vi "CmdSet_Cmd_OMAN.vi.bak.vi"(10 "cmd in":string="COLUMS 4096 ROWS 4112 PRESCAN 53 OVERSCAN 62 UTILITY /home/config/SOIAPP/DHE/util.lod TIMING_NORMAL /home/config/SOIAPP/DHE/tim_normal.lod TIMING_FOCUS /home/config/SOIAPP/DHE/tim_focus.lod READOUTMODE 3 MULTEXTEN TRUE HDR /home/config/SOIAPP/sifs.hdr SHOWIMAGE FALSE BINX 1 BINY 1 ENABLEROI FALSE ROIXCENTER 2098 ROIXSIZE 800 ROIYCENTER 2056 ROIYSIZE 400") -> (2 "cmd out":string)   [LabVIEW 2016]
panel:
  in  "bin 2":cluster{"x":i16, "y":i16}
  in  "roi 2":cluster{"xc":i16, "yc":i16, "xl":i16, "yl":i16}
  in  "bin":cluster{"x":i16, "y":i16}
  in  "roi":cluster{"xc":i16, "yc":i16, "xl":i16, "yl":i16}
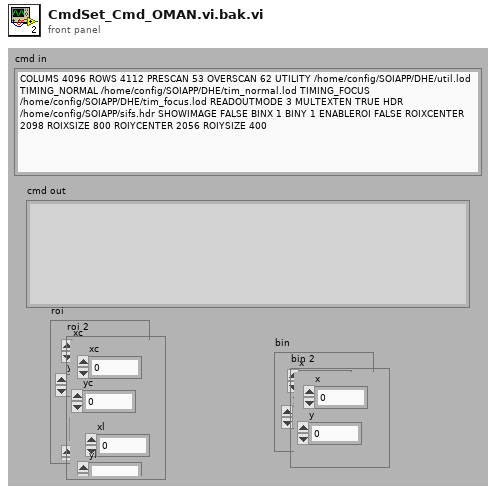
[diagram p1: front panel]
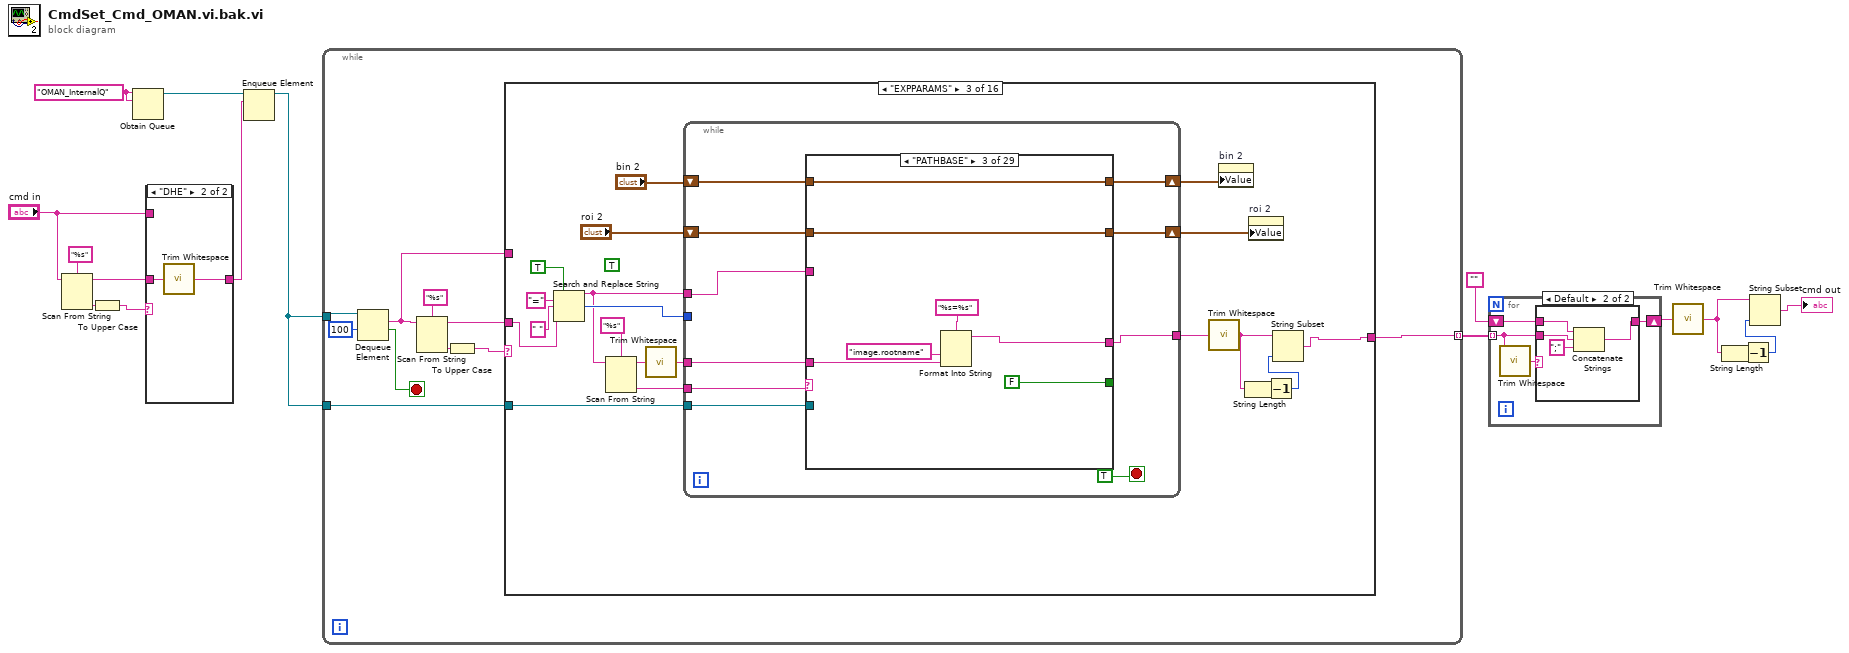
[diagram p0: block diagram]
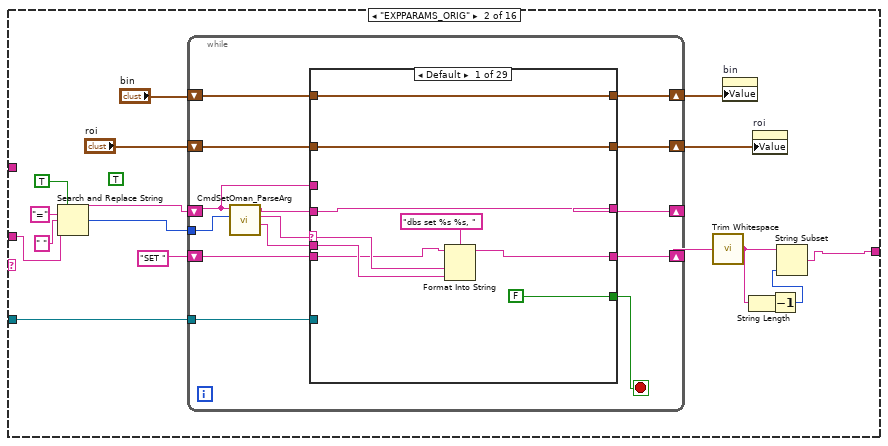
[diagram p4: hidden frame]
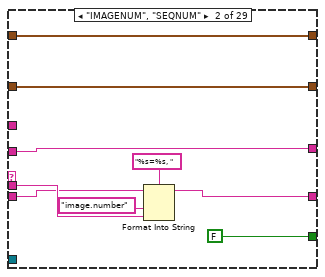
[diagram p5: hidden frame]
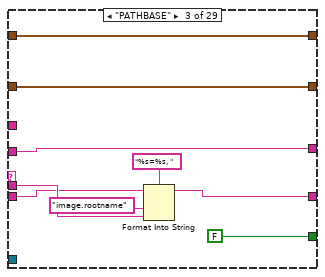
[diagram p6: hidden frame]
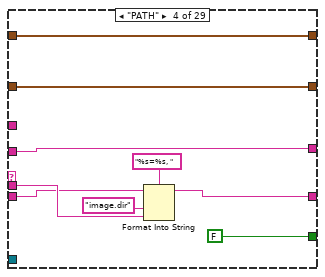
[diagram p7: hidden frame]
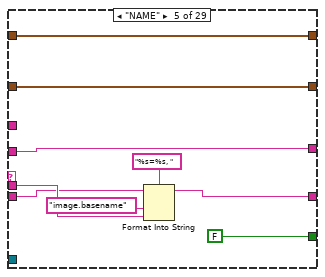
[diagram p8: hidden frame]
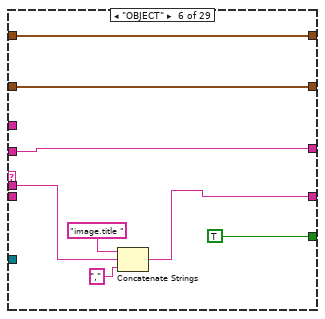
[diagram p9: hidden frame]
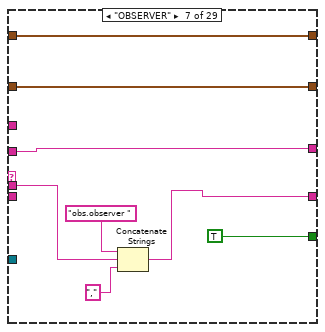
[diagram p10: hidden frame]
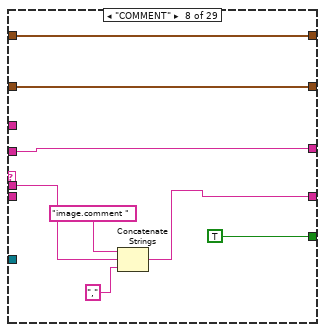
[diagram p11: hidden frame]
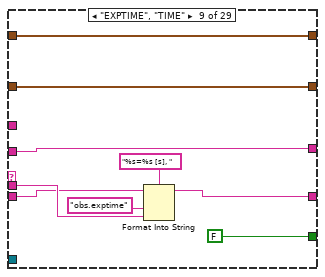
[diagram p12: hidden frame]
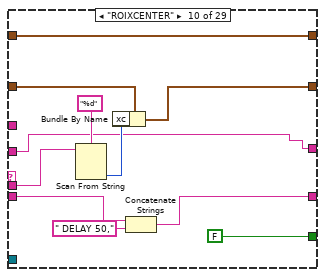
[diagram p13: hidden frame]
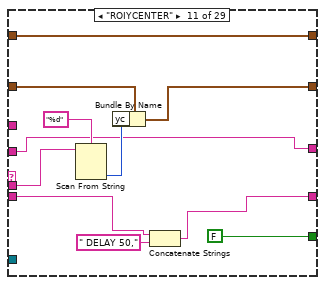
[diagram p14: hidden frame]
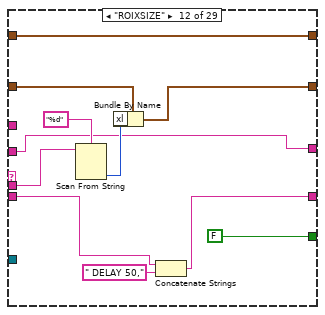
[diagram p15: hidden frame]
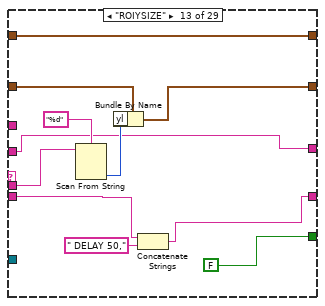
[diagram p16: hidden frame]
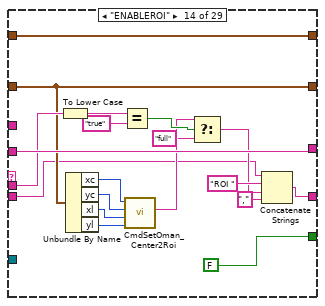
[diagram p17: hidden frame]
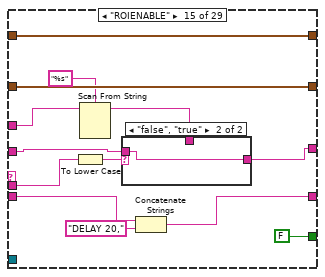
[diagram p18: hidden frame]
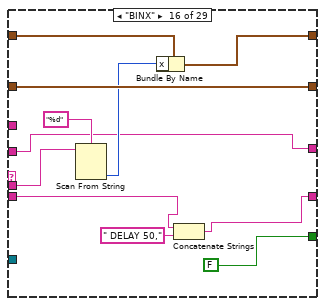
[diagram p20: hidden frame]
diagram:
  w11 = "OMAN_InternalQ" ("name (unnamed)")
  n1 = Scan From String(format string="%s", input string="cmd in") -> (remaining string=w13:string, output 1=w15:string)  [unwired: 2 in, 3 out]
  n2 = To Upper Case(1:w15) -> (0:w14:string)
  n3 = Obtain Queue(name (unnamed)=w11, element data type=w11) -> (queue out=w10:refnum<queue>)  [unwired: 3 in, 2 out]
  n4 = case shown="\"DHE\"" w14 {
    tunnel: w13 -> [_ w19]
    tunnel: [w17 w18] -> w9
    tunnel: "cmd in" -> [w17 _]
    frame Default {
    }
    frame "DHE" {
      n5 = call <vilib>:"Trim Whitespace.vi"("string"=w19) -> ("trimmed string"=w18:string)  [unwired: 1 in]
    }
  }
  n6 = Enqueue Element(queue=w10, element=w9) -> (queue out=w8:refnum<queue>)  [unwired: 1 in, 3 out]
  n7 = while {
    tunnel: w8 -> [w27]
    tunnel: w8 -> [w23]
    tunnel: [w21] -> w7 mode=indexing
    stop <- w24 stop-if-true
    n8 = Dequeue Element(queue=w27, timeout in ms (-1)=100) -> (element=w20:string, timed out?=w24:bool)  [unwired: 1 in, 2 out]
    n9 = Scan From String(format string="%s", input string=w20) -> (remaining string=w22:string, output 1=w29:string)  [unwired: 2 in, 3 out]
    n10 = To Upper Case(1:w29) -> (0:w26:string)
    n11 = case shown="\"EXPPARAMS\"" w26 {
      tunnel: [w30 w35 w344 w610 w618 "get progress" ("trimmed string") w625 w633 "pause" ("trimmed string") "resume" ("trimmed string") "DHE ASYNC SEND INIT OK" ("trimmed string") w640 "stop now" ("trimmed string") "close" ("trimmed string") "EXPOSE" ("trimmed string") "APP DELAY 50" ("trimmed string")] -> w21
      tunnel: w23 -> [_ w34 w343 _ _ _ _ _ _ _ _ _ _ _ _ _]
      tunnel: w22 -> [_ w33 w342 w604 _ _ w624 w630 _ _ _ w639 _ _ _ _]
      tunnel: w20 -> [w30 _ _ _ _ _ _ _ _ _ _ _ _ _ _ _]
      frame Default {
      }
      frame "EXPPARAMS_ORIG" {
        (unwired) TRUE ("replace all? (F)")
        n12 = Search and Replace String(replace all?=TRUE ("replace all? (F)"), input string=w33, search string="=", replace string=" " ("replace string (\"\")")) -> (result string=w32:string, number of replacements=w31:i32)  [unwired: 1 in, 5 out]
        n13 = while {
          shift-right: [w59] -> _
          shift-left: w32 -> [w49]
          shift-right: [w60] -> w43
          shift-left: "SET " -> [w58]
          shift-right: [w56] -> w38
          shift-left: "roi" -> [w57]
          shift-right: [w54] -> w37
          shift-left: "bin" -> [w55]
          tunnel: w34 -> [w53]
          tunnel: w31 -> [w48]
          stop <- w61 stop-if-true
          n14 = call "CmdSetOman_ParseArg.vi"("number of params"=w48, "args in"=w49) -> ("value"=w50:string, "key"=w51:string, "remaining args"=w52:string)  [unwired: 7 out]
          n15 = case shown="Default" w51 {
            selector: w51 -> [w67 _ _ _ _ _ _ _ _ _ _ _ _ _ _ _ _ _ _ _ _ _ _ _ _ _ w311 w321 _]
            tunnel: w50 -> [w66 w76 w85 w94 w103 w109 w117 w125 w136 w147 w158 w169 w181 w194 w207 w227 w238 _ w254 w263 _ _ _ _ _ w301 w310 w322 _]
            tunnel: [FALSE FALSE FALSE FALSE FALSE TRUE TRUE TRUE FALSE FALSE FALSE FALSE FALSE FALSE FALSE FALSE FALSE FALSE FALSE FALSE FALSE FALSE FALSE FALSE TRUE FALSE FALSE FALSE TRUE] -> w61
            tunnel: [w69 w78 w87 w96 w105 w107 w115 w123 w138 w140 w151 w162 w173 w195 w210 w218 w229 w247 w256 w265 w270 w272 w279 w286 w295 w305 w316 w327 "get status."] -> w60
            tunnel: w52 -> [w65 w75 w84 w93 w102 w113 w121 w129 w135 w143 w154 w165 w176 w201 w203 w221 w232 w245 w253 w262 w271 w278 w285 w292 w296 w306 w317 w328 _]
            tunnel: [w65 w75 w84 w93 w102 w113 w121 w129 w135 w143 w154 w165 w176 w201 w204 w221 w232 w245 w253 w262 w271 w278 w285 w292 w296 w306 w317 w328 "" ("remaining args")] -> w59
            tunnel: w58 -> [w64 w73 w82 w91 w100 _ _ _ w133 w142 w152 w163 w174 w184 w212 w219 w230 w243 w251 w260 w270 w274 w281 w288 w295 w305 w316 w327 _]
            tunnel: w57 -> [w63 w72 w81 w90 w99 w112 w120 w128 w132 w149 w160 w171 w182 w187 w214 w225 w236 w242 w250 w259 w268 w276 w283 w290 w294 w304 w315 w326 w331]
            tunnel: [w63 w72 w81 w90 w99 w112 w120 w128 w132 w148 w159 w170 w179 w187 w214 w225 w236 w242 w250 w259 w268 w276 w283 w290 w294 w304 w315 w326 w331] -> w56
            tunnel: w55 -> [w62 w71 w80 w89 w98 w111 w119 w127 w131 w144 w155 w166 w177 w197 w215 w224 w235 w241 w249 w258 w267 w275 w282 w289 w293 w303 w314 w325 w330]
            tunnel: [w62 w71 w80 w89 w98 w111 w119 w127 w131 w144 w155 w166 w177 w197 w215 w223 w234 w241 w249 w258 w267 w275 w282 w289 w293 w303 w314 w325 w330] -> w54
            tunnel: w53 -> [_ _ _ _ _ _ _ _ _ _ _ _ _ _ _ _ _ _ _ _ _ _ _ _ _ w299 w313 w324 _]
            tunnel: w49 -> [_ _ _ _ _ _ _ _ _ _ _ _ _ _ w209 _ _ _ _ _ _ _ _ _ _ _ _ _ _]
            frame Default {
              n16 = Format Into String(format string="dbs set %s %s, ", initial string=w64, w67, w66) -> (resulting string=w69:string)  [unwired: 1 in, 1 out]
            }
            frame "IMAGENUM", "SEQNUM" {
              n17 = Format Into String(format string="%s=%s, ", initial string=w73, "image.number" ("input 1"), w76) -> (resulting string=w78:string)  [unwired: 1 in, 1 out]
            }
            frame "PATHBASE" {
              n18 = Format Into String(format string="%s=%s, ", initial string=w82, "image.rootname" ("input 1"), w85) -> (resulting string=w87:string)  [unwired: 1 in, 1 out]
            }
            frame "PATH" {
              n19 = Format Into String(format string="%s=%s, ", initial string=w91, "image.dir" ("input 1"), w94) -> (resulting string=w96:string)  [unwired: 1 in, 1 out]
            }
            frame "NAME" {
              n20 = Format Into String(format string="%s=%s, ", initial string=w100, "image.basename" ("input 1"), w103) -> (resulting string=w105:string)  [unwired: 1 in, 1 out]
            }
            frame "OBJECT" {
              n21 = Concatenate Strings("image.title " ("input 1"), w109, "," ("string")) -> (w107:string)
            }
            frame "OBSERVER" {
              n22 = Concatenate Strings("obs.observer " ("input 1"), w117, "," ("string")) -> (w115:string)
            }
            frame "COMMENT" {
              n23 = Concatenate Strings("image.comment " ("input 1"), w125, "," ("string")) -> (w123:string)
            }
            frame "EXPTIME", "TIME" {
              n24 = Format Into String(format string="%s=%s [s], ", initial string=w133, "obs.exptime" ("input 1"), w136) -> (resulting string=w138:string)  [unwired: 1 in, 1 out]
            }
            frame "ROIXCENTER" {
              n25 = Scan From String(format string="%d", input string=w147) -> (output 1=w145:i32)  [unwired: 2 in, 4 out]
              n26 = Bundle By Name(cluster=w149, "xc"=w145) -> (w148:cluster{"xc":i16, "yc":i16, "xl":i16, "yl":i16})
              n27 = Concatenate Strings(w142, " DELAY 50," ("string")) -> (w140:string)
            }
            frame "ROIYCENTER" {
              n28 = Scan From String(format string="%d", input string=w158) -> (output 1=w156:i32)  [unwired: 2 in, 4 out]
              n29 = Bundle By Name(cluster=w160, "yc"=w156) -> (w159:cluster{"xc":i16, "yc":i16, "xl":i16, "yl":i16})
              n30 = Concatenate Strings(w152, " DELAY 50," ("string")) -> (w151:string)
            }
            frame "ROIXSIZE" {
              n31 = Scan From String(format string="%d", input string=w169) -> (output 1=w167:i32)  [unwired: 2 in, 4 out]
              n32 = Bundle By Name(cluster=w171, "xl"=w167) -> (w170:cluster{"xc":i16, "yc":i16, "xl":i16, "yl":i16})
              n33 = Concatenate Strings(w163, " DELAY 50," ("string")) -> (w162:string)
            }
            frame "ROIYSIZE" {
              n34 = Scan From String(format string="%d", input string=w181) -> (output 1=w178:i32)  [unwired: 2 in, 4 out]
              n35 = Bundle By Name(cluster=w182, "yl"=w178) -> (w179:cluster{"xc":i16, "yc":i16, "xl":i16, "yl":i16})
              n36 = Concatenate Strings(w174, " DELAY 50," ("string")) -> (w173:string)
            }
            frame "ENABLEROI" {
              n37 = To Lower Case(string=w194) -> (all lower case string=w192:string)
              n38 = Unbundle By Name(w187) -> ("xc"=w200:i16, "yc"=w199:i16, "xl"=w198:i16, "yl"=w186:i16)
              n39 = Equal?(x=w192, y="true") -> (x = y?=w191:bool)
              n40 = call "CmdSetOman_Center2Roi.vi"("yl"=w186, "xl"=w198, "yc"=w199, "xc"=w200) -> ("roi"=w190:string)  [unwired: 7 out]
              n41 = Select(t=w190, s=w191, f="full") -> (s? t:f=w188:string)
              n42 = Concatenate Strings(w184, "ROI " ("string"), w188, "," ("string")) -> (w195:string)
            }
            frame "ROIENABLE" {
              n43 = To Lower Case(string=w207) -> (all lower case string=w206:string)
              n44 = Scan From String(format string="%s", input string=w209) -> (remaining string=w205:string)  [unwired: 2 in, 4 out]
              n45 = case shown="\"false\", \"true\"" w206 {
                tunnel: w205 -> [w216 _]
                tunnel: [w216 w217] -> w204
                tunnel: w203 -> [_ w217]
                frame Default {
                }
                frame "false", "true" {
                }
              }
              n46 = Concatenate Strings(w212, "DELAY 20," ("string")) -> (w210:string)
            }
            frame "BINX" {
              n47 = Scan From String(format string="%d", input string=w227) -> (output 1=w222:i32)  [unwired: 2 in, 4 out]
              n48 = Bundle By Name(cluster=w224, "x"=w222) -> (w223:cluster{"x":i16, "y":i16})
              n49 = Concatenate Strings(w219, " DELAY 50," ("string")) -> (w218:string)
            }
            frame "BINY" {
              n50 = Scan From String(format string="%d", input string=w238) -> (output 1=w233:i32)  [unwired: 2 in, 4 out]
              n51 = Concatenate Strings(w230, " DELAY 50," ("string")) -> (w229:string)
              n52 = Bundle By Name(cluster=w235, "y"=w233) -> (w234:cluster{"x":i16, "y":i16})
            }
            frame "REPEATS" {
              n53 = Format Into String(format string="%s=%s, ", initial string=w243, "obs.nimages" ("input 1"), "1" ("input 2")) -> (resulting string=w247:string)  [unwired: 1 in, 1 out]
            }
            frame "MULTEXTEN" {
              n54 = Format Into String(format string="%s=%s, ", initial string=w251, "image.extensions" ("input 1"), w254) -> (resulting string=w256:string)  [unwired: 1 in, 1 out]
            }
            frame "SHOWIMAGE" {
              n55 = Format Into String(format string="%s=%s, ", initial string=w260, "obs.display" ("input 1"), w263) -> (resulting string=w265:string)  [unwired: 1 in, 1 out]
            }
            frame "COADDS", "FOWLER" {
            }
            frame "COLUMNS", "COLUMS", "HDR", "OVERSCAN", "PRESCAN", "ROWS" {
              n56 = Concatenate Strings(w274, "DELAY 20," ("string")) -> (w272:string)
            }
            frame "BUFFERSIZE", "LASTFILENAME", "TIMING_FOCUS", "TIMING_NORMAL", "UTILITY" {
              n57 = Concatenate Strings(w281, "DELAY 20," ("string")) -> (w279:string)
            }
            frame "ENABLEGRID", "FOCCENT", "FOCNUM", "FOCSTEP", "ROWPERSLICE", "ROWSPERSLICE" {
              n58 = Concatenate Strings(w288, "DELAY 20," ("string")) -> (w286:string)
            }
            frame "" {
            }
            frame "READOUTMODE" {
              n59 = case shown="\"15\", Default" w301 {
                tunnel: ["quad"] -> w300
                frame "15", Default {
                }
              }
              n60 = Concatenate Strings("macro read_" ("string"), w300) -> (w298:string)
              n61 = Enqueue Element(queue=w299, element=w298) -> ()  [unwired: 1 in, 4 out]
            }
            frame "MODE" {
              n62 = call <vilib>:"Space Constant.vi"() -> ("String"=w309:string)
              n63 = Concatenate Strings(w311, w309, w310) -> (w312:string)
              n64 = Enqueue Element(queue=w313, element=w312) -> ()  [unwired: 1 in, 4 out]
            }
            frame "OBSID", "PROPID", "PROPOSAL", "PROPOSER" {
              n65 = Format Into String(format string="FITS KEY ADD %s " ("string"), w321) -> (resulting string=w319:string)  [unwired: 2 in, 1 out]
              n66 = Concatenate Strings(w319, w322) -> (w323:string)
              n67 = Enqueue Element(queue=w324, element=w323) -> ()  [unwired: 1 in, 4 out]
            }
            frame "STATE" {
            }
          }
        }
        n68 = call <vilib>:"Trim Whitespace.vi"("string"=w43) -> ("trimmed string"=w41:string)  [unwired: 1 in]
        n69 = property on="bin" class="Clust (strict)"("Value"=w37) -> ()  [unwired: 2 in, 2 out]
        n70 = String Length(string=w41) -> (length=w42:i32)
        n71 = property on="roi" class="Clust (strict)"("Value"=w38) -> ()  [unwired: 2 in, 2 out]
        n72 = Decrement(x=w42) -> (x-1=w36:i32)
        n73 = String Subset(string=w41, length (rest)=w36) -> (substring=w35:string)  [unwired: 1 out]
      }
      frame "EXPPARAMS" {
        (unwired) TRUE ("replace all? (F)")
        n74 = Search and Replace String(replace all?=TRUE ("replace all? (F)"), input string=w342, search string="=", replace string=" " ("replace string (\"\")")) -> (result string=w340:string, number of replacements=w341:i32)  [unwired: 1 in, 5 out]
        n75 = Scan From String(format string="%s", input string=w340) -> (remaining string=w337:string, output 1=w338:string)  [unwired: 2 in, 3 out]
        n76 = call <vilib>:"Trim Whitespace.vi"("string"=w337) -> ("trimmed string"=w336:string)  [unwired: 1 in]
        n77 = while {
          shift-right: [w363] -> w347
          shift-left: "roi 2" -> [w364]
          shift-right: [w361] -> w346
          shift-left: "bin 2" -> [w362]
          tunnel: w343 -> [w360]
          tunnel: w341 -> [_]
          tunnel: w340 -> [w358]
          tunnel: w338 -> [w357]
          tunnel: w336 -> [w356]
          tunnel: [w355] -> w335
          stop <- TRUE stop-if-true
          n78 = case shown="\"PATHBASE\"" w357 {
            selector: w357 -> [w368 _ _ _ _ _ _ _ _ _ _ _ _ _ _ _ _ _ _ _ _ _ _ _ _ _ w583 w592 _]
            tunnel: w356 -> [w367 w375 w382 w390 w398 w404 w411 w418 w427 w437 w447 w457 w468 w481 w491 w509 w519 _ w533 w541 _ _ _ _ _ w574 w582 w593 _]
            tunnel: [FALSE FALSE FALSE FALSE FALSE TRUE TRUE TRUE FALSE FALSE FALSE FALSE FALSE FALSE FALSE FALSE FALSE FALSE FALSE FALSE FALSE FALSE FALSE FALSE TRUE FALSE FALSE FALSE TRUE] -> _
            tunnel: [w370 w377 w384 w392 w400 w402 w409 w416 w429 w431 w441 w451 w461 w482 w494 w501 w511 w527 w535 w543 w548 w549 w555 w561 w569 w578 w588 w598 "get status."] -> w355
            tunnel: w364 -> [w366 w373 w380 w387 w395 w407 w414 w421 w424 w439 w449 w459 w469 w474 w498 w507 w517 w523 w530 w538 w546 w553 w559 w565 w568 w577 w587 w597 w601]
            tunnel: [w366 w373 w380 w387 w395 w407 w414 w421 w424 w438 w448 w458 w466 w474 w498 w507 w517 w523 w530 w538 w546 w553 w559 w565 w568 w577 w587 w597 w601] -> w363
            tunnel: w362 -> [w365 w372 w379 w386 w394 w406 w413 w420 w423 w434 w444 w454 w464 w484 w499 w506 w516 w522 w529 w537 w545 w552 w558 w564 w567 w576 w586 w596 w600]
            tunnel: [w365 w372 w379 w386 w394 w406 w413 w420 w423 w434 w444 w454 w464 w484 w499 w505 w515 w522 w529 w537 w545 w552 w558 w564 w567 w576 w586 w596 w600] -> w361
            tunnel: w360 -> [_ _ _ _ _ _ _ _ _ _ _ _ _ _ _ _ _ _ _ _ _ _ _ _ _ w572 w585 w595 _]
            tunnel: w358 -> [_ _ _ _ _ _ _ _ _ _ _ _ _ _ w493 _ _ _ _ _ _ _ _ _ _ _ _ _ _]
            frame Default {
              n79 = Format Into String(format string="dbs set %s %s", w368, w367) -> (resulting string=w370:string)  [unwired: 2 in, 1 out]
            }
            frame "IMAGENUM", "SEQNUM" {
              n80 = Format Into String(format string="%s=%s", "image.number" ("input 1"), w375) -> (resulting string=w377:string)  [unwired: 2 in, 1 out]
            }
            frame "PATHBASE" {
              n81 = Format Into String(format string="%s=%s", "image.rootname" ("input 1"), w382) -> (resulting string=w384:string)  [unwired: 2 in, 1 out]
            }
            frame "PATH" {
              n82 = Format Into String(format string="%s=%s, ", "image.dir" ("input 1"), w390) -> (initial string=w388:string, resulting string=w392:string)  [unwired: 1 in, 1 out]
            }
            frame "NAME" {
              n83 = Format Into String(format string="%s=%s, ", "image.basename" ("input 1"), w398) -> (initial string=w396:string, resulting string=w400:string)  [unwired: 1 in, 1 out]
            }
            frame "OBJECT" {
              n84 = Concatenate Strings("image.title " ("input 1"), w404, "," ("string")) -> (w402:string)
            }
            frame "OBSERVER" {
              n85 = Concatenate Strings("obs.observer " ("input 1"), w411, "," ("string")) -> (w409:string)
            }
            frame "COMMENT" {
              n86 = Concatenate Strings("image.comment " ("input 1"), w418, "," ("string")) -> (w416:string)
            }
            frame "EXPTIME", "TIME" {
              n87 = Format Into String(format string="%s=%s [s], ", "obs.exptime" ("input 1"), w427) -> (initial string=w425:string, resulting string=w429:string)  [unwired: 1 in, 1 out]
            }
            frame "ROIXCENTER" {
              n88 = Scan From String(format string="%d", input string=w437) -> (output 1=w435:i32)  [unwired: 2 in, 4 out]
              n89 = Bundle By Name(cluster=w439, "xc"=w435) -> (w438:cluster{"xc":i16, "yc":i16, "xl":i16, "yl":i16})
              n90 = Concatenate Strings(" DELAY 50," ("string")) -> (w431:string, w433:string)
            }
            frame "ROIYCENTER" {
              n91 = Scan From String(format string="%d", input string=w447) -> (output 1=w445:i32)  [unwired: 2 in, 4 out]
              n92 = Bundle By Name(cluster=w449, "yc"=w445) -> (w448:cluster{"xc":i16, "yc":i16, "xl":i16, "yl":i16})
              n93 = Concatenate Strings(" DELAY 50," ("string")) -> (w441:string, w442:string)
            }
            frame "ROIXSIZE" {
              n94 = Scan From String(format string="%d", input string=w457) -> (output 1=w455:i32)  [unwired: 2 in, 4 out]
              n95 = Bundle By Name(cluster=w459, "xl"=w455) -> (w458:cluster{"xc":i16, "yc":i16, "xl":i16, "yl":i16})
              n96 = Concatenate Strings(" DELAY 50," ("string")) -> (w451:string, w452:string)
            }
            frame "ROIYSIZE" {
              n97 = Scan From String(format string="%d", input string=w468) -> (output 1=w465:i32)  [unwired: 2 in, 4 out]
              n98 = Bundle By Name(cluster=w469, "yl"=w465) -> (w466:cluster{"xc":i16, "yc":i16, "xl":i16, "yl":i16})
              n99 = Concatenate Strings(" DELAY 50," ("string")) -> (w461:string, w462:string)
            }
            frame "ENABLEROI" {
              n100 = To Lower Case(string=w481) -> (all lower case string=w479:string)
              n101 = Unbundle By Name(w474) -> ("xc"=w487:i16, "yc"=w486:i16, "xl"=w485:i16, "yl"=w473:i16)
              n102 = Equal?(x=w479, y="true") -> (x = y?=w478:bool)
              n103 = call "CmdSetOman_Center2Roi.vi"("yl"=w473, "xl"=w485, "yc"=w486, "xc"=w487) -> ("roi"=w477:string)  [unwired: 7 out]
              n104 = Select(t=w477, s=w478, f="full") -> (s? t:f=w475:string)
              n105 = Concatenate Strings("ROI " ("string"), w475, "," ("string")) -> (w482:string, w471:string)
            }
            frame "ROIENABLE" {
              n106 = To Lower Case(string=w491) -> (all lower case string=w490:string)
              n107 = Scan From String(format string="%s", input string=w493) -> (remaining string=w489:string)  [unwired: 2 in, 4 out]
              n108 = case shown="Default" w490 {
                tunnel: w489 -> [w500 _]
                tunnel: [w500 _] -> _
                frame Default {
                }
                frame "false", "true" {
                }
              }
              n109 = Concatenate Strings("DELAY 20," ("string")) -> (w494:string, w496:string)
            }
            frame "BINX" {
              n110 = Scan From String(format string="%d", input string=w509) -> (output 1=w504:i32)  [unwired: 2 in, 4 out]
              n111 = Bundle By Name(cluster=w506, "x"=w504) -> (w505:cluster{"x":i16, "y":i16})
              n112 = Concatenate Strings(" DELAY 50," ("string")) -> (w501:string, w502:string)
            }
            frame "BINY" {
              n113 = Scan From String(format string="%d", input string=w519) -> (output 1=w514:i32)  [unwired: 2 in, 4 out]
              n114 = Concatenate Strings(" DELAY 50," ("string")) -> (w511:string, w512:string)
              n115 = Bundle By Name(cluster=w516, "y"=w514) -> (w515:cluster{"x":i16, "y":i16})
            }
            frame "REPEATS" {
              n116 = Format Into String(format string="%s=%s, ", "obs.nimages" ("input 1"), "1" ("input 2")) -> (initial string=w524:string, resulting string=w527:string)  [unwired: 1 in, 1 out]
            }
            frame "MULTEXTEN" {
              n117 = Format Into String(format string="%s=%s, ", "image.extensions" ("input 1"), w533) -> (initial string=w531:string, resulting string=w535:string)  [unwired: 1 in, 1 out]
            }
            frame "SHOWIMAGE" {
              n118 = Format Into String(format string="%s=%s, ", "obs.display" ("input 1"), w541) -> (initial string=w539:string, resulting string=w543:string)  [unwired: 1 in, 1 out]
            }
            frame "COADDS", "FOWLER" {
            }
            frame "COLUMNS", "COLUMS", "HDR", "OVERSCAN", "PRESCAN", "ROWS" {
              n119 = Concatenate Strings("DELAY 20," ("string")) -> (w549:string, w551:string)
            }
            frame "BUFFERSIZE", "LASTFILENAME", "TIMING_FOCUS", "TIMING_NORMAL", "UTILITY" {
              n120 = Concatenate Strings("DELAY 20," ("string")) -> (w555:string, w557:string)
            }
            frame "ENABLEGRID", "FOCCENT", "FOCNUM", "FOCSTEP", "ROWPERSLICE", "ROWSPERSLICE" {
              n121 = Concatenate Strings("DELAY 20," ("string")) -> (w561:string, w563:string)
            }
            frame "" {
            }
            frame "READOUTMODE" {
              n122 = case shown="\"15\", Default" w574 {
                tunnel: ["quad"] -> w573
                frame "15", Default {
                }
              }
              n123 = Concatenate Strings("macro read_" ("string"), w573) -> (w571:string)
              n124 = Enqueue Element(queue=w572, element=w571) -> ()  [unwired: 1 in, 4 out]
            }
            frame "MODE" {
              n125 = call <vilib>:"Space Constant.vi"() -> ("String"=w581:string)
              n126 = Concatenate Strings(w583, w581, w582) -> (w584:string)
              n127 = Enqueue Element(queue=w585, element=w584) -> ()  [unwired: 1 in, 4 out]
            }
            frame "OBSID", "PROPID", "PROPOSAL", "PROPOSER" {
              n128 = Format Into String(format string="FITS KEY ADD %s " ("string"), w592) -> (resulting string=w590:string)  [unwired: 2 in, 1 out]
              n129 = Concatenate Strings(w590, w593) -> (w594:string)
              n130 = Enqueue Element(queue=w595, element=w594) -> ()  [unwired: 1 in, 4 out]
            }
            frame "STATE" {
              (unwired) "" ("remaining args")
            }
          }
        }
        n131 = call <vilib>:"Trim Whitespace.vi"("string"=w335) -> ("trimmed string"=w350:string)  [unwired: 1 in]
        n132 = property on="bin 2" class="Clust (strict)"("Value"=w346) -> ()  [unwired: 2 in, 2 out]
        n133 = String Length(string=w350) -> (length=w351:i32)
        n134 = property on="roi 2" class="Clust (strict)"("Value"=w347) -> ()  [unwired: 2 in, 2 out]
        n135 = Decrement(x=w351) -> (x-1=w345:i32)
        n136 = String Subset(string=w350, length (rest)=w345) -> (substring=w344:string)  [unwired: 1 out]
      }
      frame "ENABLEROI", "ROI", "ROIENABLE" {
        n137 = Scan From String(format string="%s", input string=w604) -> (output 1=w608:string)  [unwired: 2 in, 4 out]
        n138 = property on="roi" class="Clust (strict)"() -> ("Value"=w612:cluster{"xc":i16, "yc":i16, "xl":i16, "yl":i16})  [unwired: 2 in, 2 out]
        n139 = Unbundle By Name(w612) -> ("xc"=w615:i16, "yc"=w614:i16, "xl"=w613:i16, "yl"=w605:i16)
        n140 = call "CmdSetOman_Center2Roi.vi"("yl"=w605, "xl"=w613, "yc"=w614, "xc"=w615) -> ("roi"=w607:string)  [unwired: 7 out]
        n141 = case shown="\"\", \"on\", \"true\", \"yes\"" w608 {
          tunnel: w607 -> [_ w617]
          tunnel: ["full" ("roi") w617] -> w606
          frame Default {
          }
          frame "", "on", "true", "yes" {
          }
        }
        n142 = Concatenate Strings("SET ROI " ("string"), w606) -> (w610:string)
      }
      frame "BINNING" {
        n143 = property on="bin" class="Clust (strict)"() -> ("Value"=w622:cluster{"x":i16, "y":i16})  [unwired: 2 in, 2 out]
        n144 = Unbundle By Name(w622) -> ("x"=w621:i16, "y"=w620:i16)
        n145 = Format Into String(format string="set binning %d %d", w621, w620) -> (resulting string=w618:string)  [unwired: 2 in, 1 out]
      }
      frame "EXP_PROG" {
      }
      frame "MODE" {
        n146 = Scan From String(format string="%s", input string=w624) -> (output 1=w626:string)  [unwired: 2 in, 4 out]
        n147 = case shown="Default" w626 {
          tunnel: ["macro mode_normal" ("trimmed string") "macro mode_focus " ("trimmed string")] -> w625
          frame Default {
          }
          frame "FOCUS" {
          }
        }
      }
      frame "STATUS" {
        n148 = Scan From String(format string="%s", input string=w630) -> (output 1=w631:string)  [unwired: 2 in, 4 out]
        n149 = case shown="\"EXP_PROG\", \"EXP_PROG2\"" w631 {
          tunnel: ["" ("trimmed string") "get progress" ("trimmed string")] -> w633
          frame Default {
          }
          frame "EXP_PROG", "EXP_PROG2" {
          }
        }
      }
      frame "PAUSEEXP" {
      }
      frame "RESUMEEXP" {
      }
      frame "INITCTR" {
      }
      frame "DRIVER" {
        n150 = Scan From String(format string="%s", input string=w639) -> (output 1=w642:string)  [unwired: 2 in, 4 out]
        n151 = To Lower Case(string=w642) -> (all lower case string=w641:string)
        n152 = case shown="\"open\"" w641 {
          tunnel: ["close" ("trimmed string") "init" ("trimmed string")] -> w640
          frame Default {
          }
          frame "open" {
          }
        }
      }
      frame "ABORTEXP" {
      }
      frame "RELEASECTR" {
      }
      frame "FIRST_EXPOSE" {
      }
      frame "SEQFIN" {
      }
    }
  }
  n153 = for {
    tunnel: w7 -> [w651] mode=indexing
    shift-right: [w652] -> w2
    shift-left: "" -> [w653]
    n154 = call <vilib>:"Trim Whitespace.vi"("string"=w651) -> ("trimmed string"=w650:string)  [unwired: 1 in]
    n155 = case shown="Default" w650 {
      tunnel: w651 -> [_ w658]
      tunnel: w653 -> [w654 w656]
      tunnel: [w654 w655] -> w652
      frame "", "SE" {
      }
      frame Default {
        n156 = Concatenate Strings(w656, w658, ";" ("string")) -> (w655:string)
      }
    }
  }
  n157 = call <vilib>:"Trim Whitespace.vi"("string"=w2) -> ("trimmed string"=w1:string)  [unwired: 1 in]
  n158 = String Length(string=w1) -> (length=w5:i32)
  n159 = Decrement(x=w5) -> (x-1=w4:i32)
  n160 = String Subset(string=w1, length (rest)=w4) -> (substring=→"cmd out":string)  [unwired: 1 out]
